vi "plot theory_energy.vi"() -> ()   [LabVIEW 2016]
panel:
  out "XY Graph":cluster{dbl[], dbl[]}[](graph)
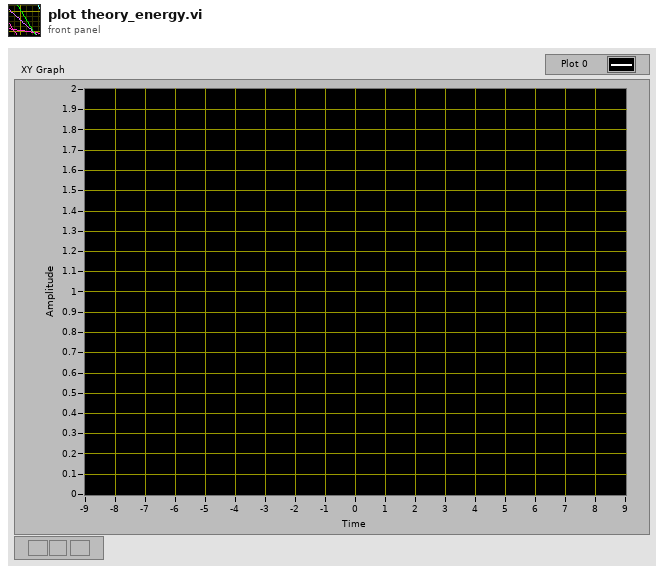
[diagram p1: front panel]
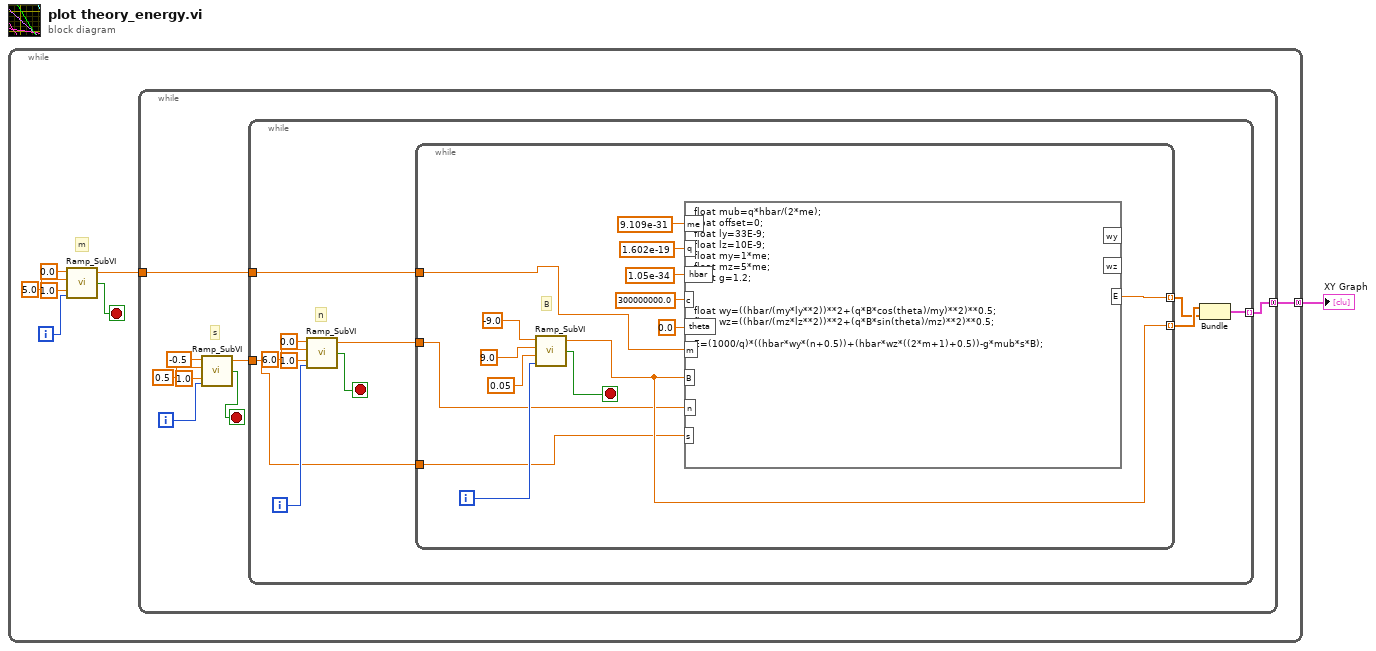
[diagram p0: block diagram]
diagram:
  n1 = while {
    tunnel: [w8] -> w1 mode=concatenating
    i -> [w4]
    stop <- w3 stop-if-true
    # "m"
    n2 = call <userlib>:"Ramp_SubVI.vi"("index"=w4, "step"=1.0, "end"=5.0, "start"=0.0) -> ("Stop?"=w3:bool, "Numeric"=w2:dbl)  [unwired: 1 in]
    n3 = while {
      tunnel: [w16] -> w8 mode=concatenating
      tunnel: w2 -> [w9]
      i -> [w10]
      stop <- w12 stop-if-true
      # "s"
      n4 = call <userlib>:"Ramp_SubVI.vi"("index"=w10, "step"=1.0, "end"=0.5, "start"=-0.5) -> ("Stop?"=w12:bool, "Numeric"=w11:dbl)  [unwired: 1 in]
      n5 = while {
        tunnel: [w19] -> w16 mode=indexing
        tunnel: w11 -> [w18]
        tunnel: w9 -> [w17]
        i -> [w24]
        stop <- w23 stop-if-true
        # "n"
        n6 = call <userlib>:"Ramp_SubVI.vi"("index"=w24, "step"=1.0, "end"=6.0, "start"=0.0) -> ("Stop?"=w23:bool, "Numeric"=w22:dbl)  [unwired: 1 in]
        n7 = while {
          tunnel: w22 -> [w30]
          tunnel: [w32] -> w20 mode=indexing
          tunnel: [w31] -> w21 mode=indexing
          tunnel: w18 -> [w29]
          tunnel: w17 -> [w28]
          i -> [w35]
          stop <- w34 stop-if-true
          # "B"
          n8 = call <userlib>:"Ramp_SubVI.vi"("index"=w35, "step"=0.05, "end"=9.0, "start"=-9.0) -> ("Stop?"=w34:bool, "Numeric"=w31:dbl)  [unwired: 1 in]
          n9 = formula code="float mub=q*hbar/(2*me);\nfloat offset=0;\nfloat ly=33E-9;\nfloat lz=10E-9;\nfloat my=1*me;\nfloat mz=5*me;\nfloat g=1.2;\n\n\nfloat wy=((hbar/(my*ly**2))**2+(q*B*cos(theta)/my)**2)**0.5;\nfloat wz=((hbar/(mz*lz**2))**2+(q*B*sin(theta)/mz)**2)**0.5;\n\nE=(1000/q)*((hbar*wy*(n+0.5))+(hbar*wz*((2*m+1)+0.5))-g*mub*s*B);"("me"=9.109e-31 ("input variable"), "q"=1.602e-19 ("input variable"), "hbar"=1.05e-34 ("input variable"), "c"=300000000.0 ("input variable"), "B"=w31, "theta"=0.0 ("input variable"), "n"=w30, "m"=w28, "s"=w29) -> ("E"=w32:dbl)  [unwired: 2 out]
        }
        n10 = Bundle(w21, w20) -> (w19:cluster{dbl[], dbl[]})  [unwired: 1 in]
      }
    }
  }
  "XY Graph" <- w1
